vi "Set_Frames.vi"(8 "error in (no error)":errorcluster, 10 "Frames":i32, 11 "Abstract_CCD in":refnum<class "Abstract_CCD.lvclass">) -> (0 "error out":errorcluster, 3 "Abstract_CCD out":refnum<class "Abstract_CCD.lvclass">)   [LabVIEW 2014, in "Abstract_CCD.lvclass"]
uses:
  Abstract_CCD.lvclass
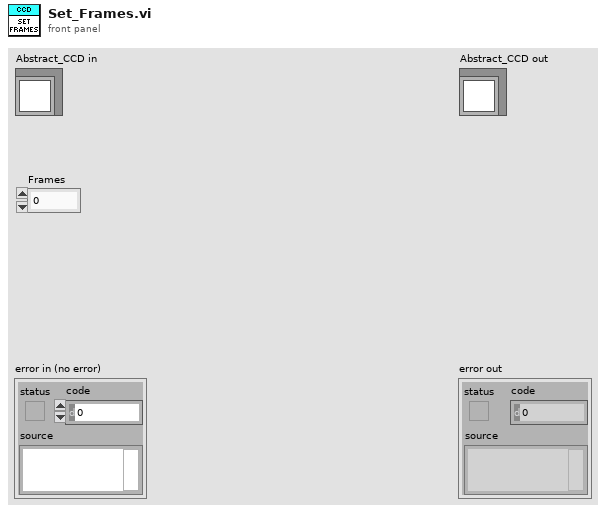
[diagram p1: front panel]
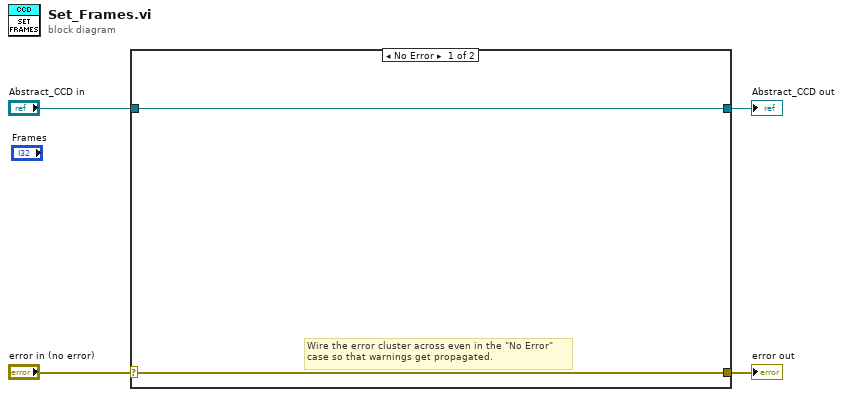
[diagram p0: block diagram]
diagram:
  n1 = case shown="No Error" "error in (no error)" {
    selector: "error in (no error)" -> [w5 w8]
    tunnel: [w5 w8] -> w3
    tunnel: [w6 w7] -> w1
    tunnel: "Abstract_CCD in" -> [w6 w7]
    frame No Error {
      # "Wire the error cluster across even in the \"No Error\"\ncase so that warnings get propagated."
    }
    frame Error {
    }
  }
  "error out" <- w3
  "Abstract_CCD out" <- w1
